vi "Convertion in Json for test.vi"() -> ()   [LabVIEW 2020]
uses:
  Commun VI/TypeDef/Commande Test/Commande Parameter Flash_Jlink.ctl
  Commun VI/TypeDef/Command Power_Supply/Parameter Power_Supply.ctl
  Class/Power_Supply/Power_Supply (Default)/Power_Supply (Default).lvclass
  Commun VI/TypeDef/Commande Test/Commande Parameter Flash_.AVRDUDEctl.ctl
  Commun VI/TypeDef/Command Power_Supply/Data_Write_Power_Supply.ctl
  Class/JSON API/JSON Value/Set from JSON string.vi
  Class/JSON API/Variant JSON/Variant to JSON.vi
  Class/JSON API/JSON Value/Get Item by name array.vi
  Class/JSON API/JSON Value/JSON Value.lvclass
  Class/JSON API/Get Polymorphic/JSON GetSet.lvlib
  Class/JSON API/Variant JSON/Variant JSON.lvlib
  Commun VI/Library Commun.lvlib
panel:
  out "données":T1={"Device_Addr"="USB0::0x1AB1::0x09C4::DM3R194602503::INSTR", "Current"=0.0, "Channel"=0, "Voltage"=0.0, " Class Power_Supply"=refnum}
  in  "?":T2={"Path FW"=path "C:/Users/ngarcin/Altyor/QUALITY-ALTYOR - Documents/Test equipment management/Standard Test bench/Standard Test bench dev/Software/Test bench/Standard TB/JLink/JLink.exe", "Working Directory"=path "", "Device"="", "Frequency"="", "Connection_Type"=""}
  out "<JSON>":string
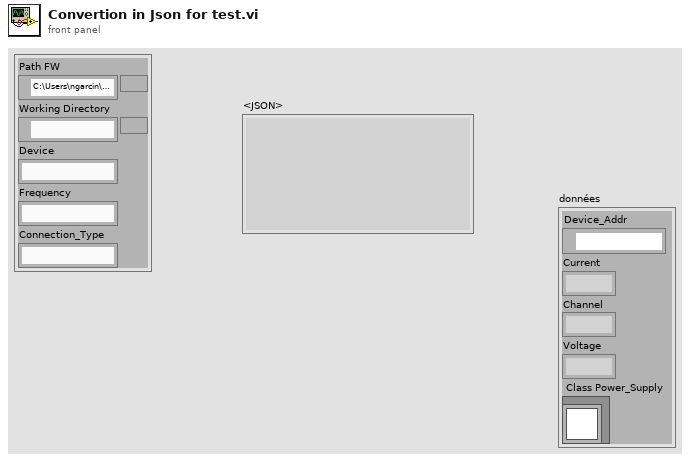
[diagram p1: front panel]
types:
  T1 = typedef "Library Commun.lvlib/Parameter Power_Supply.ctl" = cluster{"Device_Addr":refnum<visa-resource-name>, "Current":dbl, "Channel":i32, "Voltage":dbl, " Class Power_Supply":refnum<class "Power_Supply (Default).lvclass">}
  T2 = typedef "Library Commun.lvlib/Commande Parameter Flash_Jlink.ctl" = cluster{"Path FW":path, "Working Directory":path, "Device":string, "Frequency":string, "Connection_Type":string}
  T3 = cluster{"Commande Type":string, "Command ID":string, "Data":string, "Error":string}
  T4 = cluster{"Rate":u8, "Nb Sample":u8, "Voltage Max":dbl, "Voltage Min":dbl, "Input terminal Configuration":string, "Channel":u8[], "Nb Data_To_Read":i16}
  T5 = cluster{"Information_Operator":string, "Path_Picture":path, "Timeout (ms)":u64, "Weight":dbl}
  T6 = cluster{"Weight":dbl, "Front":enum16{"Amount", "Descending"}}
  T7 = cluster{"Connection":string, "Database":string[], "Table":string, "Columm":string, "Value":string}
  T8 = cluster{"Path File InstallCode":path, "Store With CRC":bool}
  T9 = cluster{"Bootloader path":path, "Firmware path":path, "Security path":path, "Serial number":path, "commander path":path}
  T10 = cluster{"Center Freq (MHz)":dbl, "Freq Span (MHz)":dbl, "Ref Level (dBm)":dbl, "Threshold (dBm)":dbl}
  T11 = cluster{"Class Parsing Data":string, "TimeOut":u16, "R-org":string, "Func":string}
  T12 = typedef "Library Commun.lvlib/Data_Write_Power_Supply.ctl" = enum16{"Enable Channel", "Disable Channel"}
  T13 = cluster{"Global_File_Signed":path, "Key_File":path, "FW_File_Signed":path, "Working Directory":path}
  T14 = cluster{"Device":string, "Working Directory":path, "FW_File":path, "Key_File":path, "FW_File_Signed":path}
  T15 = cluster{"Path_File_Key_Pub":path, "Device":string, "Function":enum16{"Sign", "Command"}}
  T16 = cluster{"Working Directory":path, "Device":string}
  T17 = cluster{"Working Directory":path, "Argument":string, "Path FW":path, "Extension File":string}
  T18 = cluster{"Path FW":path, "Working Directory":path, "Argument":string}
  T19 = cluster{"TimeOut":u16, "R-org":string, "Frame Type":enum16{"Teach IN", "Normal Mode"}}
  T20 = cluster{"Path file Json":path, "Server":string, "Profile":string}
  T21 = cluster{"Time On":u8, "Time Off":u8, "Relay":i32}
  T22 = cluster{"Number Prog":string, "Test Number":u16, "Timeout":u16}
  T23 = cluster{"Class SN":string, "Protocol":string, "Product Number":string}
  T24 = cluster{"Address Device":refnum<visa-resource-name>, "Baud Rate":u32, "Data Bit":u16, "stop bits (10: 1 bit)":u16, "parity (0:none)":enum16{"None", "Odd", "Even", "Mark", "Space"}, "flow control (0:none)":u16, "termination char ":u8, "Enable Termination":bool}
  T25 = cluster{"Frame Read":string, "Frame received":bool, "Frame NOk":bool}
  T26 = cluster{"Device_Com_Port":string, "Address Board":string}
  T27 = cluster{"Information_Operator":string, "Ok_Button_Visible":bool, "Picture":path, "Timeout (ms)":u16, "Function":enum16{"Write", "Read"}, "Line":u8, "Port":u8}
  T28 = cluster{"Information_Operator":string, "Ok_Button_Visible":bool, "Path_Picture":path}
  T29 = cluster{"Information_Operator":string, "Ok_Button_Visible":bool}
  T30 = typedef "Commande Parameter Flash_.AVRDUDEctl.ctl" = cluster{"Path FW ":path, "Working Directory":path, "Device":string, "Frequency":string}
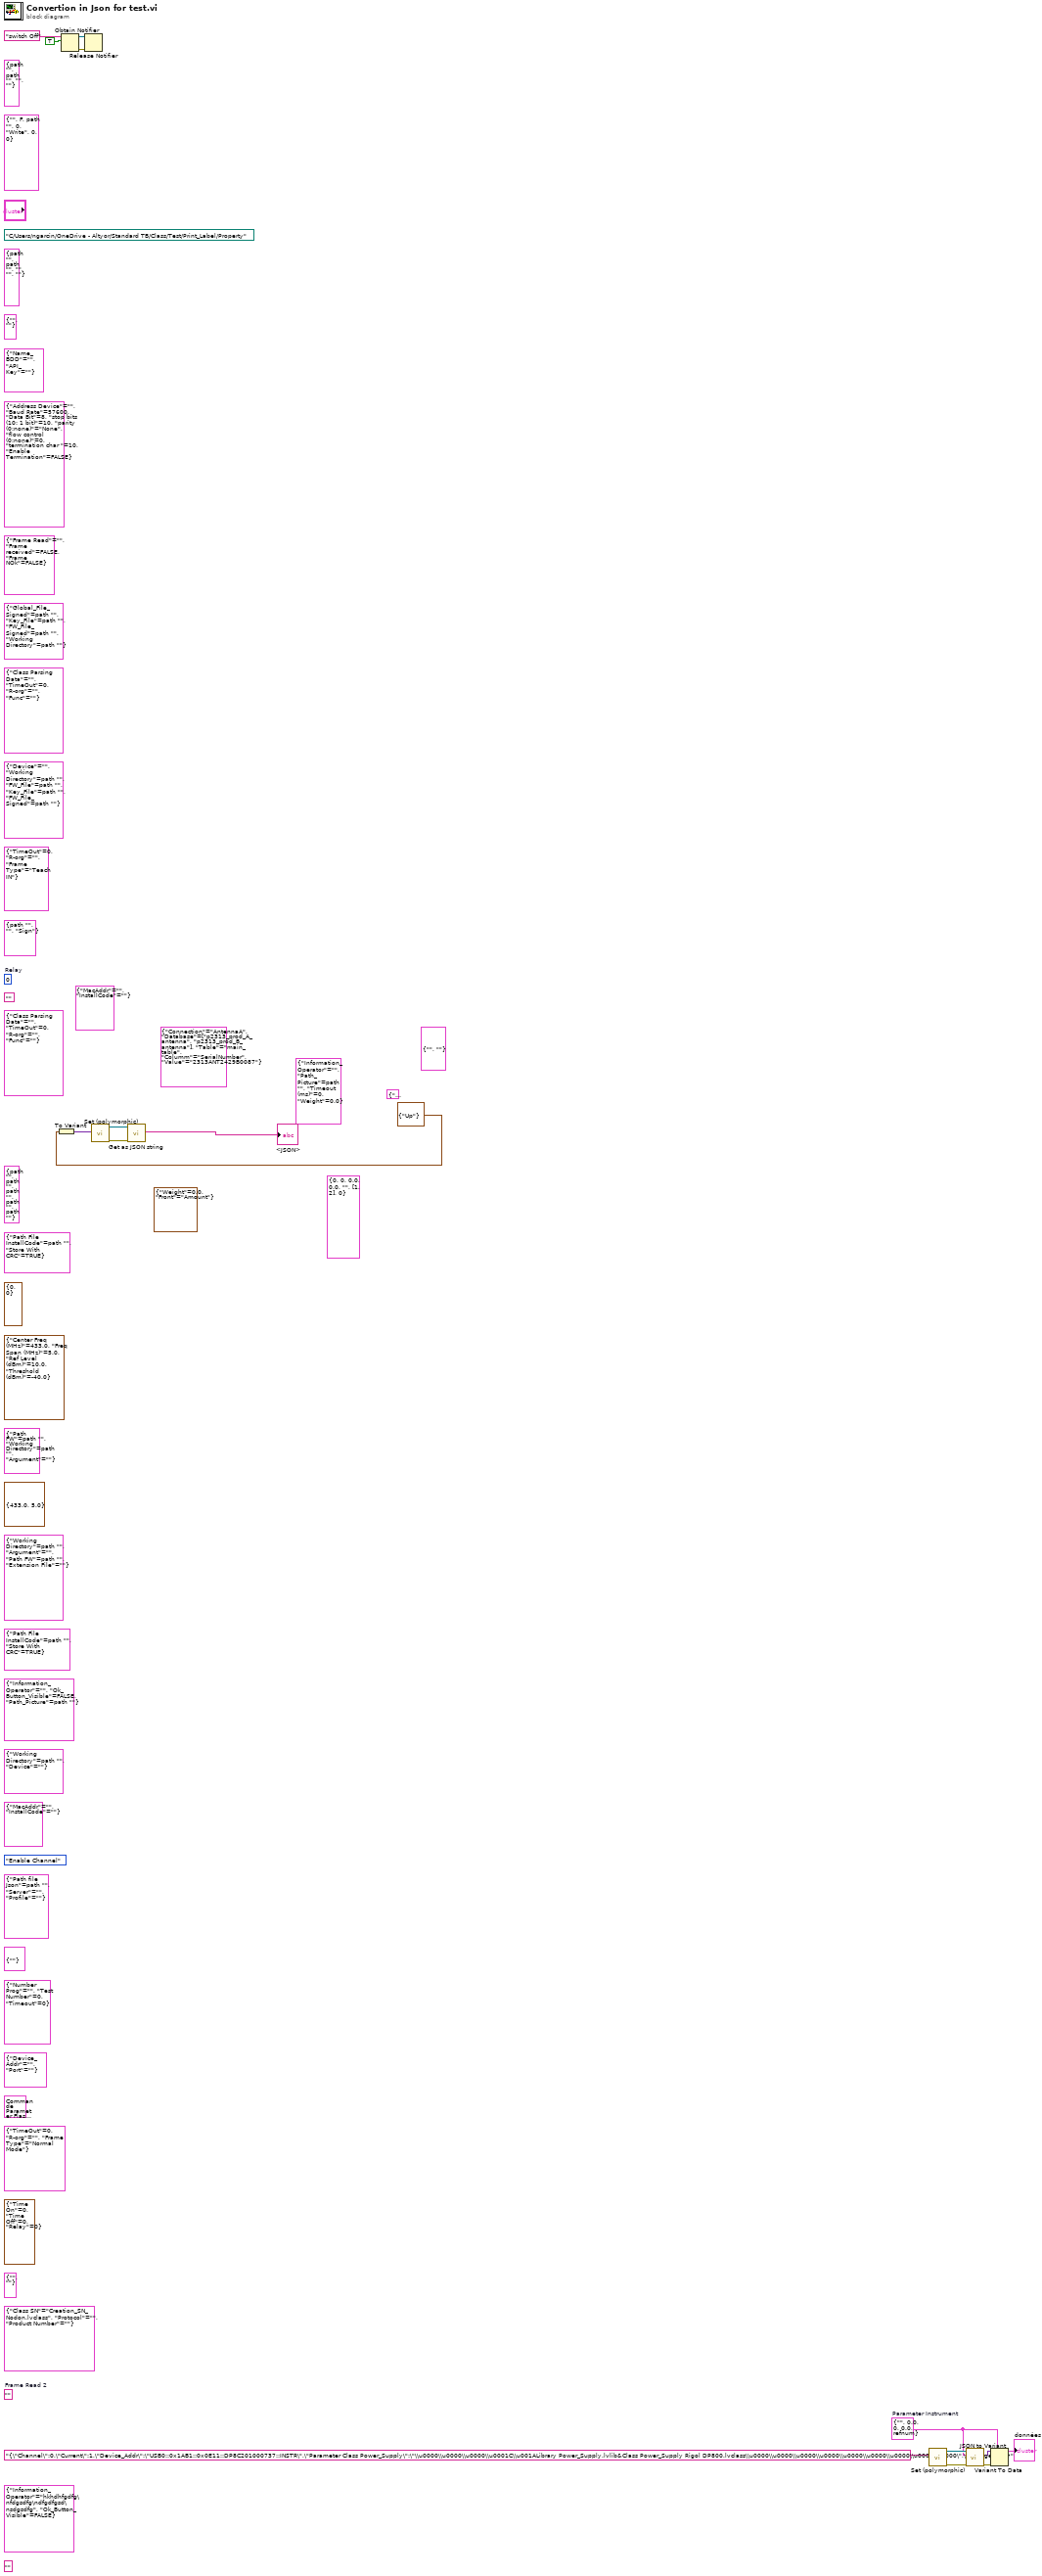
[diagram p0: block diagram]
diagram:
  (unwired) cluster{"Switch":string, "Type":string} {"Switch"="", "Type"=""}
  (unwired) T3 {"Commande Type"="", "Command ID"="", "Data"="", "Error"=""}
  (unwired) T4 {"Rate"=0, "Nb Sample"=0, "Voltage Max"=0.0, "Voltage Min"=0.0, "Input terminal Configuration"="", "Channel"=[1, 2], "Nb Data_To_Read"=0} ("Parameter")
  (unwired) T5 {"Information_Operator"="", "Path_Picture"=path "", "Timeout (ms)"=0, "Weight"=0.0} ("Cluster des données privées de classe")
  (unwired) T6 {"Weight"=0.0, "Front"=enum."Amount"}
  (unwired) cluster{"MacAddr":string, "InstallCode":string} {"MacAddr"="", "InstallCode"=""}
  (unwired) T7 {"Connection"="AntennaA", "Database"=["p2313_prod_A_antenna", "p2313_prod_B_antenna"], "Table"="main_table", "Columm"="SerialNumber", "Value"="2313ANT2429B0087"} ("Parameter")
  (unwired) T8 {"Path File InstallCode"=path "", "Store With CRC"=TRUE}
  (unwired) T9 {"Bootloader path"=path "", "Firmware path"=path "", "Security path"=path "", "Serial number"=path "", "commander path"=path ""} ("Cluster des données privées de classe")
  (unwired) cluster{"Line":u8, "Port":u8} {"Line"=0, "Port"=0} ("Cluster des données privées de classe")
  (unwired) T10 {"Center Freq (MHz)"=433.0, "Freq Span (MHz)"=5.0, "Ref Level (dBm)"=10.0, "Threshold (dBm)"=-40.0} ("Cluster des données privées de classe")
  (unwired) cluster{"Frenquency":dbl, "Power":dbl} {"Frenquency"=433.0, "Power"=5.0} ("Parameter")
  (unwired) T11 {"Class Parsing Data"="", "TimeOut"=0, "R-org"="", "Func"=""}
  (unwired) Data_Write_Power_Supply."Enable Channel" ("Function")
  (unwired) cluster{"PRCE":string} {"PRCE"=""}
  (unwired) cluster{"MacAddr":string, "InstallCode":string} {"MacAddr"="", "InstallCode"=""}
  (unwired) T13 {"Global_File_Signed"=path "", "Key_File"=path "", "FW_File_Signed"=path "", "Working Directory"=path ""} ("Cluster des données privées de classe")
  (unwired) T14 {"Device"="", "Working Directory"=path "", "FW_File"=path "", "Key_File"=path "", "FW_File_Signed"=path ""} ("Cluster")
  (unwired) T15 {"Path_File_Key_Pub"=path "", "Device"="", "Function"=enum."Sign"} ("Cluster des données privées de classe")
  (unwired) T16 {"Working Directory"=path "", "Device"=""} ("Cluster")
  (unwired) T17 {"Working Directory"=path "", "Argument"="", "Path FW"=path "", "Extension File"=""} ("Cluster")
  (unwired) T18 {"Path FW"=path "", "Working Directory"=path "", "Argument"=""} ("Cluster")
  (unwired) T8 {"Path File InstallCode"=path "", "Store With CRC"=TRUE}
  (unwired) T19 {"TimeOut"=0, "R-org"="", "Frame Type"=enum."Teach IN"}
  (unwired) T20 {"Path file Json"=path "", "Server"="", "Profile"=""}
  (unwired) T21 {"Time On"=0, "Time Off"=0, "Relay"=0} ("Cluster des données privées de classe")
  (unwired) T19 {"TimeOut"=0, "R-org"="", "Frame Type"=enum."Normal Mode"}
  (unwired) cluster{"Device_Addr":string, "Port":string} {"Device_Addr"="", "Port"=""} ("Parameter")
  (unwired) cluster{"Device_Addr":string, "Port":string} {"Device_Addr"="", "Port"=""} ("Parameter")
  (unwired) T22 {"Number Prog"="", "Test Number"=0, "Timeout"=0} ("Parameter")
  (unwired) ""  # Frame Read 2
  (unwired) T23 {"Class SN"="Creation_SN_Nodon.lvclass", "Protocol"="", "Product Number"=""}
  (unwired) T11 {"Class Parsing Data"="", "TimeOut"=0, "R-org"="", "Func"=""}
  (unwired) T24 {"Address Device"="", "Baud Rate"=57600, "Data Bit"=8, "stop bits (10: 1 bit)"=10, "parity (0:none)"=enum."None", "flow control (0:none)"=0, "termination char "=10, "Enable Termination"=FALSE} ("Parameter")
  (unwired) ""
  (unwired) T25 {"Frame Read"="", "Frame received"=FALSE, "Frame NOk"=FALSE}
  (unwired) path "C:/Users/ngarcin/OneDrive - Altyor/Standard TB/Class/Test/Print_Label/Property" ("Path_Picture")
  (unwired) T26 {"Device_Com_Port"="", "Address Board"=""} ("Parameter")
  (unwired) cluster{"Name_BDD":string, "API_Key":string} {"Name_BDD"="", "API_Key"=""} ("Parameter")
  (unwired) T27 {"Information_Operator"="", "Ok_Button_Visible"=FALSE, "Picture"=path "", "Timeout (ms)"=0, "Function"=enum."Write", "Line"=0, "Port"=0} ("Cluster des données privées de classe")
  (unwired) T28 {"Information_Operator"="", "Ok_Button_Visible"=FALSE, "Path_Picture"=path ""}
  (unwired) T29 {"Information_Operator"="hkhdhfgdfg\nfdgsdfg\ndfgdfgsd\nsdgsdfg", "Ok_Button_Visible"=FALSE}
  (unwired) T30 {"Path FW "=path "", "Working Directory"=path "", "Device"="", "Frequency"=""}
  (unwired) T2 {"Path FW"=path "", "Working Directory"=path "", "Device"="", "Frequency"="", "Connection_Type"=""}
  (unwired) 0  # Relay
  (unwired) "" ("FW Version")
  w3 = T1 {"Device_Addr"="", "Current"=0.0, "Channel"=0, "Voltage"=0.0, " Class Power_Supply"=refnum}  # Parameter Instrument
  (unwired) T30 {"Path FW "=path "C:/Users/ngarcin/Altyor/P2265-SCHNEIDER ELECTRIC-ZIGBEE KNX BRIDGE - PROJECT DOCUMENTS/10-MANUFACTURING PRODUCT/TEST BENCH/Test bench FW files/attiny10_firmware.hex", "Working Directory"=path "C:/Users/ngarcin/Altyor/QUALITY-ALTYOR - Documents/Test equipment management/Standard Test bench/Standard Test bench dev/Class/Test/Flash_AVRDUDE/AVRDUDE", "Device"="t10", "Frequency"="93.75"}
  n1 = To Variant(anything=cluster{"State":enum16{"Up", "Down", "Stop"}} {"State"=enum."Up"}) -> (Variant=w16:variant)
  n2 = Obtain Notifier(name (unnamed)="switch Off" ("nom (aucun)"), notification data type=TRUE) -> (notifier out=w9:refnum<notifier>, error out=w10:errorcluster)  [unwired: 2 in, 1 out]
  n3 = Release Notifier(notifier=w9, error in (no error)=w10) -> ()  [unwired: 1 in, 3 out]
  n4 = call-poly "Set (polymorphic).vi"("Variant"=w16) -> ("error out"=w14:errorcluster, "JSON Value out"=w15:refnum<class "JSON Value.lvclass">)  [unwired: 9 in]
  n5 = call "Get as JSON string.vi"("error in (no error)"=w14, "JSON Value in"=w15) -> ("<JSON>"=→"<JSON>":string)  [unwired: 8 in, 1 out]
  n6 = call-poly "Set (polymorphic).vi"("JSON stream"="{\"Channel\":0,\"Current\":1,\"Device_Addr\":\"USB0::0x1AB1::0x0E11::DP8C201000737::INSTR\",\"Parameter Class Power_Supply\":\"\\u0000\\u0000\\u0000\\u0001C\\u001ALibrary Power_Supply.lvlib&Class Power_Supply Rigol DP800.lvclass\\u0000\\u0000\\u0000\\u0000\\u0000\\u0000\\u0000\\u0000\\u0000\",\"Voltage\":24}") -> ("error out"=w6:errorcluster, "JSON Value out"=w8:refnum<class "JSON Value.lvclass">)  [unwired: 8 in, 1 out]
  n7 = call "JSON to Variant.vi"("error in (no error)"=w6, "Variant (Data Type)"=w3, "JSON Value"=w8) -> ("error out"=w7:errorcluster, "Variant out"=w5:variant)  [unwired: 7 in]
  n8 = Variant To Data(error in=w7, type=w3, Variant=w5) -> (data=→"données":T1)  [unwired: 1 out]
